vi "LogiLABsimu.vi"() -> ()   [LabVIEW 2013]
uses:
  <vilib>/Waveform/DWDTOps.llb/DWDT Analog to Digital.vi
  <vilib>/measure/NI_MABase.lvlib
panel:
  in  "On/Off":bool
  in  "Digital Output Number":T1(radio)
  out "Digital Waveform Graph":digitalwaveform(graph)
  in  "Analog Output Number":enum32{"1", " 2", " 3", " 4", " 5", " 6"}(radio)
  out "Waveform Graph":dynamicdata(graph)
  # "LogiLab | By Ali Can oçal & Fouad Asil | supervisor : Assist. Prof. Dr. Murat AKSOY |2016"
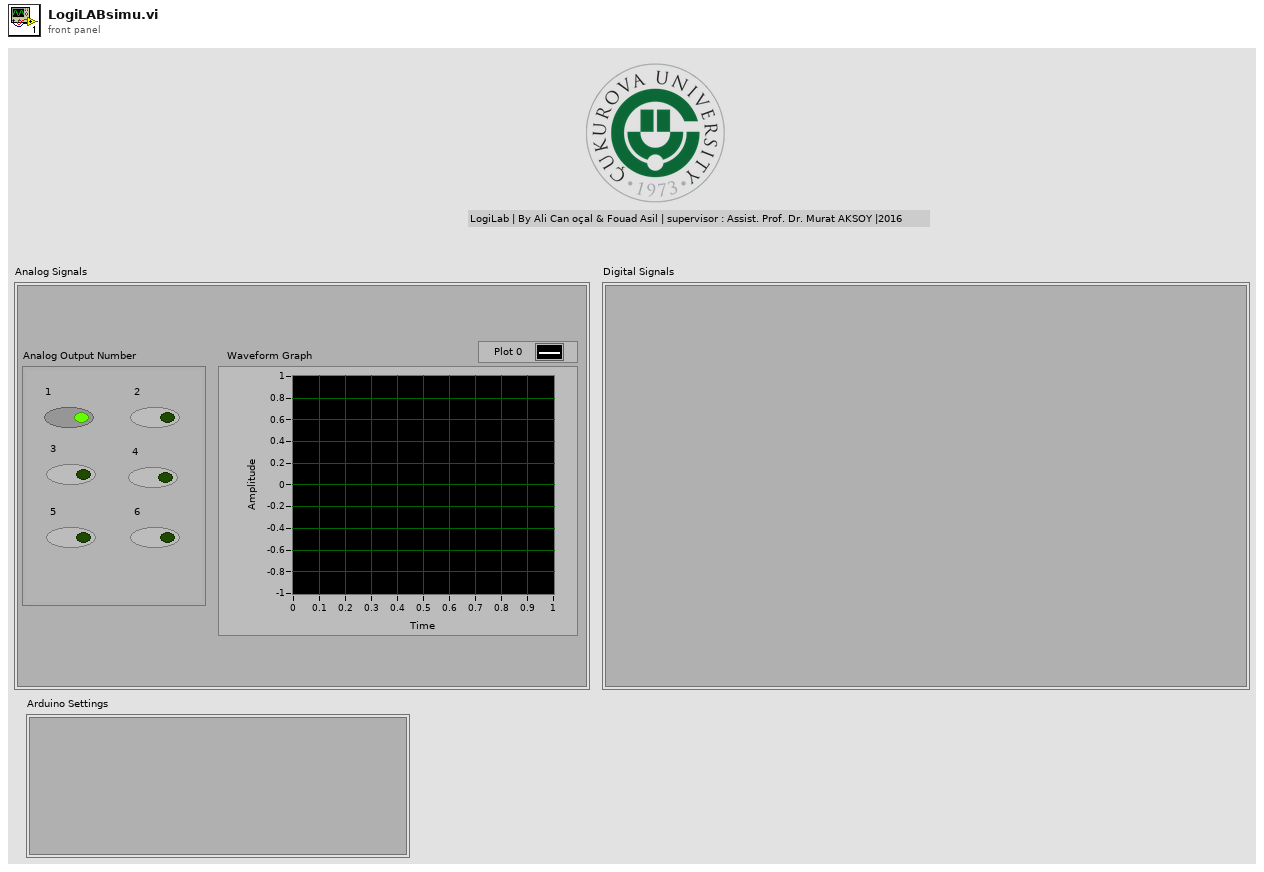
[diagram p1: front panel]
types:
  T1 = enum32{"1", " 2", " 3", " 4", " 5", " 6", " 7", " 8"}
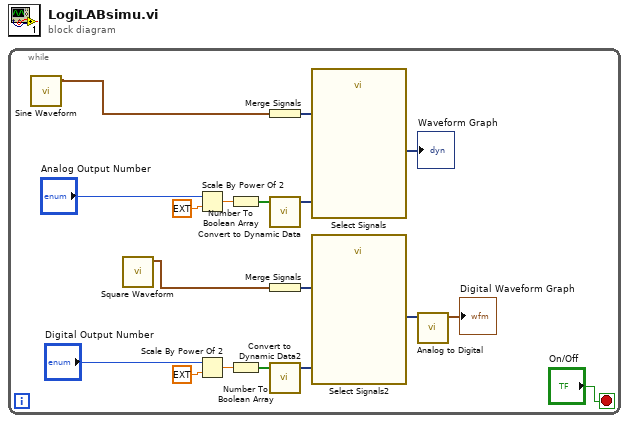
[diagram p0: block diagram]
diagram:
  n1 = while {
    stop <- "On/Off" stop-if-true
    n2 = call <vilib>:"Sine Waveform.vi"() -> ("signal out"=w1:waveform(dbl))  [unwired: 10 in, 1 out]
    n3 = call <vilib>:"Square Waveform.vi"() -> ("signal out"=w2:waveform(dbl))  [unwired: 10 in, 1 out]
    n4 = Scale By Power Of 2(n="Analog Output Number", x=ext 1.0) -> (x*2^n=w14:ext)
    n5 = Scale By Power Of 2(n="Digital Output Number", x=ext 1.0) -> (x*2^n=w8:ext)
    n6 = Number To Boolean Array(number=w14) -> (Boolean array=w13:bool[])
    n7 = Number To Boolean Array(number=w8) -> (Boolean array=w7:bool[])
    n8 = Merge Signals(w1) -> (w17:dynamicdata)
    n9 = call "Convert to Dynamic Data"("Array"=w13) -> ("Dynamic Data Type"=w12:dynamicdata)  [unwired: 3 in]
    n10 = Merge Signals(w2) -> (w5:dynamicdata)
    n11 = call "Convert to Dynamic Data2"("Array"=w7) -> ("Dynamic Data Type"=w6:dynamicdata)  [unwired: 3 in]
    n12 = call "Select Signals"("Selector Input"=w12, "Signals"=w17) -> ("Signal Out"=→"Waveform Graph":dynamicdata)  [unwired: 8 in, 1 out]
    n13 = call "Select Signals2"("Selector Input"=w6, "Signals"=w5) -> ("Signal Out"=w4:dynamicdata)  [unwired: 8 in, 1 out]
    n14 = call-poly <vilib>:"Analog to Digital.vi"("analog waveform"=w4) -> ("digital waveform"=→"Digital Waveform Graph":digitalwaveform)  [unwired: 7 in, 3 out]
  }
